vi "Add Bus Controller.vi"(6 "acyclic frame names":string[](array[string]), 8 "error in":errorcluster, 11 "port in":T1 format="%.0x") -> (0 "error out":errorcluster, 2 "bus controller":T1 format="%.0x", 3 "port out":T1 format="%.0x")   [LabVIEW 2020, in "AIM MIL-STD-1553 Scripting.lvlib"]
doc: "Adds a bus controller to the <b>port in</b> in the custom device system definition and returns the newly added <b>bus controller</b> reference."
uses:
  AIM MIL-STD-1553 Scripting.lvlib
  <vilib>/NI VeriStand/Custom Device API/Custom Device API.lvlib
  Constants.vi
  <vilib>/NI VeriStand/Custom Device API/Custom Device Item Ref.ctl
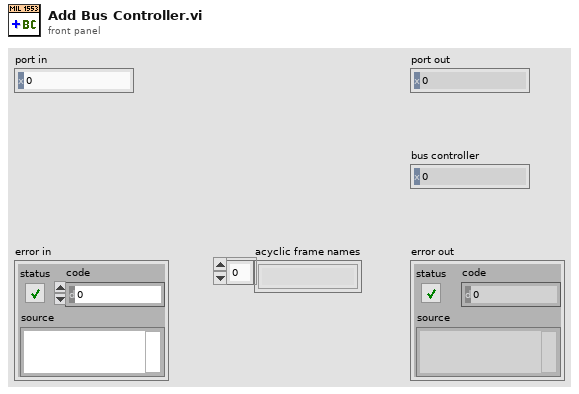
[diagram p1: front panel]
types:
  T1 = typedef "Custom Device API.lvlib/Custom Device Item Ref.ctl" = u64
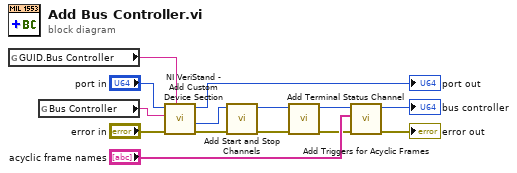
[diagram p0: block diagram]
diagram:
  n1 = global read "Constants.vi" "GUID.Bus Controller"() -> (w14:string)
  n2 = global read "Constants.vi" "Bus Controller"() -> (w10:string)
  n3 = call <vilib>:"NI VeriStand - Add Custom Device Section.vi"("GUID (Default Section)"=w14, "error in (no error)"="error in", "Section Name"=w10, "Parent Ref in"="port in") -> ("error out"=w9:errorcluster, "Section Ptr"=w6:T1, "Parent Ref out"=→"port out":T1)  [unwired: 4 in, 1 out]
  n4 = call "Add Start and Stop Channels.vi"("error in"=w9, "terminal in"=w6) -> ("error out"=w3:errorcluster, "terminal out"=w4:T1)  [unwired: 6 in, 2 out]
  n5 = call "Add Terminal Status Channel.vi"("error in"=w3, "terminal in"=w4) -> ("error out"=w1:errorcluster, "terminal out"=w2:T1)  [unwired: 7 in, 1 out]
  n6 = call "Add Triggers for Acyclic Frames.vi"("error in"=w1, "acyclic frame names"="acyclic frame names", "bus controller in"=w2) -> ("error out"=→"error out":errorcluster, "bus controller out"=→"bus controller":T1)  [unwired: 7 in]
